vi "DeviceClose.vi"(0 "Multimeter":refnum<visa-resource-name>, 1 "Commutator":refnum<visa-resource-name>, 2 "Power Source":refnum<visa-resource-name>) -> ()   [LabVIEW 2021]
panel:
  out "error out":errorcluster
  in  "error in":errorcluster
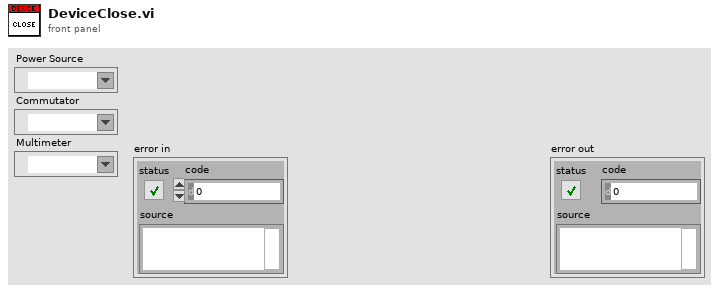
[diagram p1: front panel]
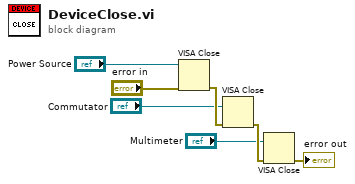
[diagram p0: block diagram]
diagram:
  n1 = VISA Close(VISA resource name="Power Source", error in (no error)="error in") -> (error out=w6:errorcluster)
  n2 = VISA Close(VISA resource name="Commutator", error in (no error)=w6) -> (error out=w5:errorcluster)
  n3 = VISA Close(VISA resource name="Multimeter", error in (no error)=w5) -> (error out=→"error out":errorcluster)
